vi "DAQ_Settings.vi"(6 "Channel":tag, 10 "rate":dbl=1000.0 format="%0.2f", 11 "sample mode":i32(ring)=10123 items=["Finite Samples"=10178, "Continuous Samples"=10123, "Hardware Timed Single Point"=12522]) -> (0 "error out":errorcluster, 2 "task out":refnum<k21>)   [LabVIEW 2023, in "Test_Libraries.lvlib"]
uses:
  Proyecto/Test_Libraries.lvlib
  <vilib>/DAQmx/create/channels.llb/DAQmx Create Channel (AI-Voltage-Basic).vi
  <vilib>/DAQmx/configure/timing.llb/DAQmx Timing (Sample Clock).vi
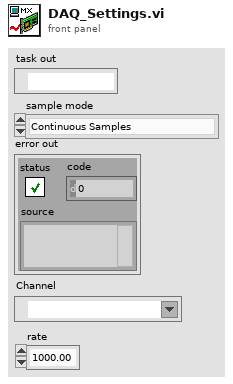
[diagram p1: front panel]
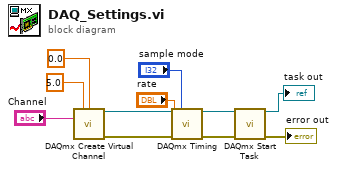
[diagram p0: block diagram]
diagram:
  n1 = call-poly <vilib>:"DAQmx Create Virtual Channel.vi"("maximum value"=5.0, "minimum value"=0.0, "physical channels"="Channel") -> ("task out"=w8:refnum<k21>, "error out"=w9:errorcluster)  [unwired: 11 in]
  n2 = call-poly <vilib>:"DAQmx Timing.vi"("task/channels in"=w8, "sample mode"="sample mode", "rate"="rate", "error in"=w9) -> ("task out"=w10:refnum<k21>, "error out"=w11:errorcluster)  [unwired: 10 in]
  n3 = call <vilib>:"DAQmx Start Task.vi"("task/channels in"=w10, "error in"=w11) -> ("task out"=→"task out":refnum<k21>, "error out"=→"error out":errorcluster)  [unwired: 12 in]
